vi "SetColor.vi"(8 "error in (no error)":errorcluster, 10 "Color":u32(colorbox), 11 "ColorRGBA in":refnum<class "ColorRGBA.lvclass">) -> (0 "error out":errorcluster, 3 "ColorRGBA out":refnum<class "ColorRGBA.lvclass">)   [LabVIEW 2021, in "Picture2D.lvlib" / "ColorRGBA.lvclass"]
uses:
  ColorRGBA.lvclass
  ColorRGB/ColorRGB.lvclass
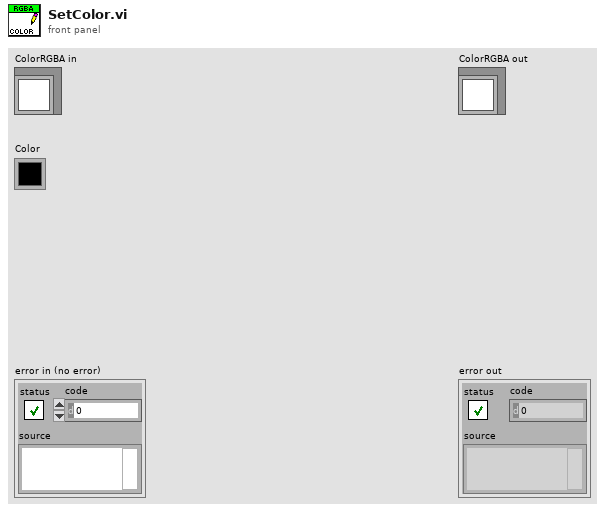
[diagram p1: front panel]
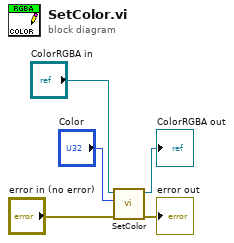
[diagram p0: block diagram]
diagram:
  n1 = call-parent "SetColor.vi"("error in (no error)"="error in (no error)", "Color"="Color", "ColorRGB in"="ColorRGBA in") -> ("error out"=→"error out":errorcluster, "ColorRGB out"=→"ColorRGBA out":refnum<class "ColorRGBA.lvclass">)  [unwired: 7 in]
